vi "UAPublishStructure.vi"(8 "error in (no error)":errorcluster, 10 "OPC UA server refnum in":refnum<k21>, 11 "Server config info":T1) -> (0 "error out":errorcluster, 2 "OPC UA server refnum out":refnum<k21>, 3 "Server config info (dup)":T1)   [LabVIEW 2014, in "OPCUA XML.lvlib"]
uses:
  OPCUA XML.lvlib
  DEF-Server Config Data.ctl
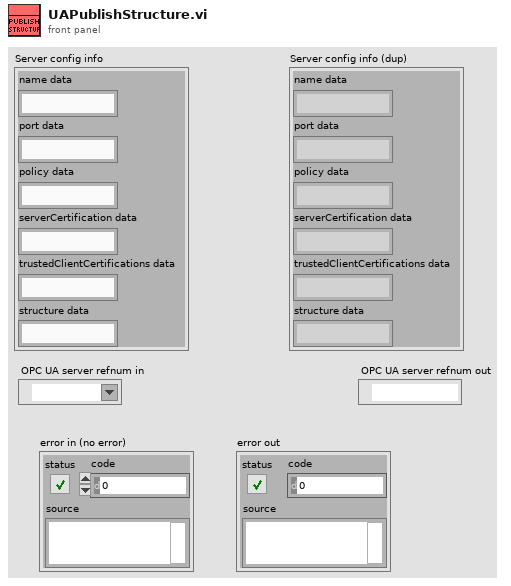
[diagram p1: front panel]
types:
  T1 = typedef "OPCUA XML.lvlib/DEF-Server Config Data.ctl" = cluster{"name data":string, "port data":string, "policy data":string, "serverCertification data":string, "trustedClientCertifications data":string, "structure data":string}
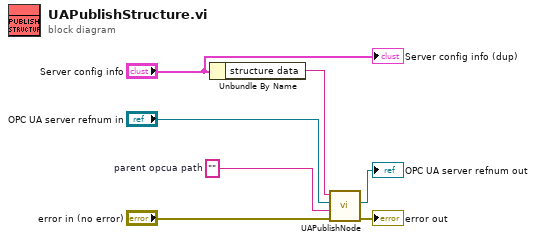
[diagram p0: block diagram]
diagram:
  w5 = ""  # parent opcua path
  n1 = Unbundle By Name("Server config info") -> ("structure data"=w6:string)
  n2 = call "UAPublishNode.vi"("error in (no error)"="error in (no error)", "parent opcua path"=w5, "OPC UA server refnum in"="OPC UA server refnum in", "content"=w6) -> ("error out"=→"error out":errorcluster, "OPC UA server refnum out"=→"OPC UA server refnum out":refnum<k21>)  [unwired: 6 in]
  "Server config info (dup)" <- "Server config info"
